vi "Add Pulse Measurement.vi"(8 "error in (no error)":errorcluster, 10 "Item Names":string[](array[string]), 11 "Monitor-Pulse in":refnum<class "Monitor-Pulse.lvclass">) -> (0 "error out":errorcluster, 3 "Monitor-Pulse out":refnum<class "Monitor-Pulse.lvclass">)   [LabVIEW 2015, in "Monitor-Pulse.lvclass"]
uses:
  Monitor-Pulse.lvclass
  Monitor-Pulse.lvclass/Monitor-Pulse.ctl
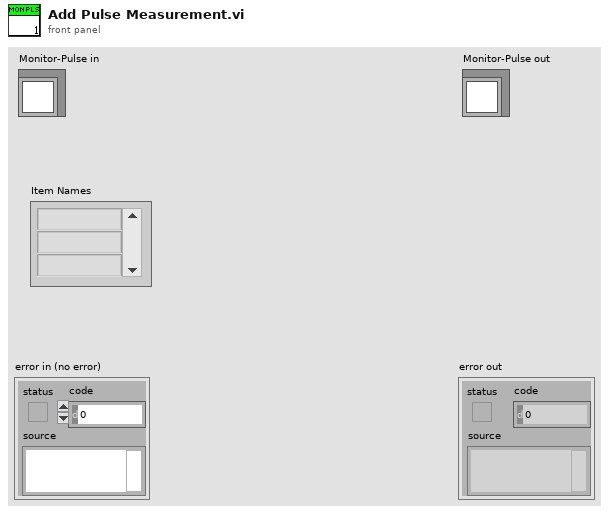
[diagram p1: front panel]
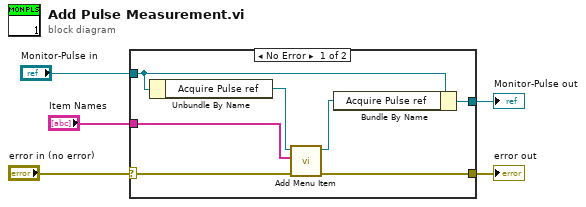
[diagram p0: block diagram]
diagram:
  n1 = case shown="No Error" "error in (no error)" {
    selector: "error in (no error)" -> [w7 w14]
    tunnel: [w9 w14] -> w4
    tunnel: [w8 w13] -> w2
    tunnel: "Monitor-Pulse in" -> [w11 w13]
    tunnel: "Item Names" -> [w6 _]
    frame No Error {
      n2 = Unbundle By Name(w11) -> ("Acquire Pulse ref"=w12:refnum<vi>)
      n3 = call "Add Menu Item.vi"("error in (no error)"=w7, "Item Names"=w6, "Queed Listbox ref"=w12) -> ("error out"=w9:errorcluster, "Queed Listbox ref out"=w10:refnum<vi>)  [unwired: 6 in, 1 out]
      n4 = Bundle By Name(cluster=w11, "Acquire Pulse ref"=w10) -> (w8:refnum<class "Monitor-Pulse.lvclass">)
    }
    frame Error {
    }
  }
  "error out" <- w4
  "Monitor-Pulse out" <- w2
